vi "PEM SubVI.vi"(0 "VISA Refnum in":refnum<visa-resource-name>, 2 "Nuevo Retardo":dbl min=0.0 max=19999.900390625 step=0.10000000149011612 format="%.3f", 3 "Nueva Long. de Onda (nm)":dbl min=0.0 max=19999.9 step=0.1 format="%.1f", 5 "Cambiar Retardo PEM":bool, 7 "Cambiar L. Onda PEM":bool, 9 "Leer Frecuencia":bool, 11 "error in (no error)":errorcluster, 13 "Reiniciar Valores":bool, 14 "stop":bool) -> (4 "VISA Refnum out":refnum<visa-resource-name>, 6 "Longitud de onda (nm)":dbl format="%_5f", 8 "Retardo":dbl format="%_5f", 10 "Frecuencia":dbl format="%_5f", 15 "error out":errorcluster)   [LabVIEW 2016]
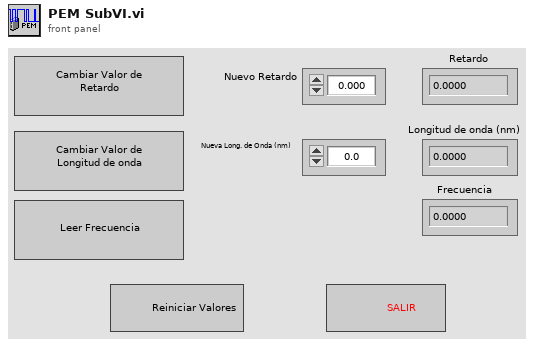
[diagram p1: front panel]
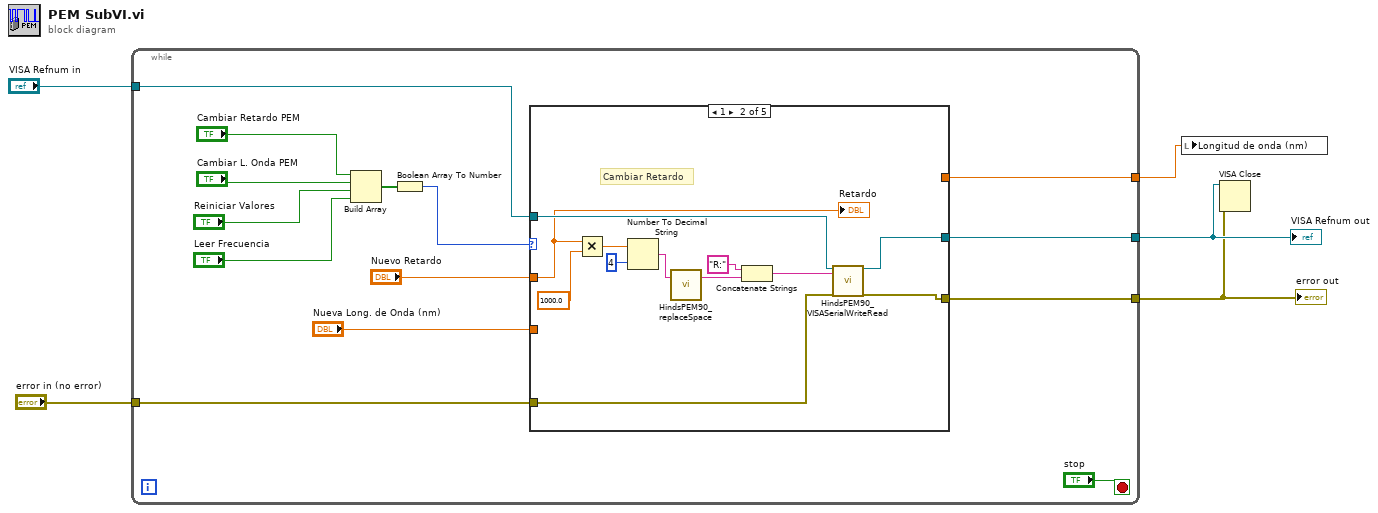
[diagram p0: block diagram]
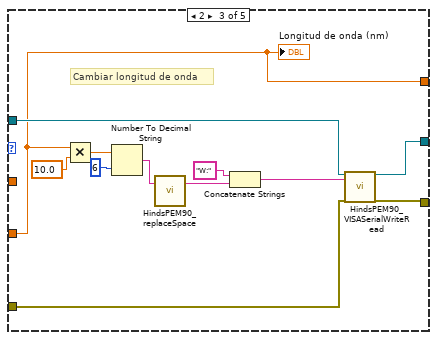
[diagram p3: hidden frame]
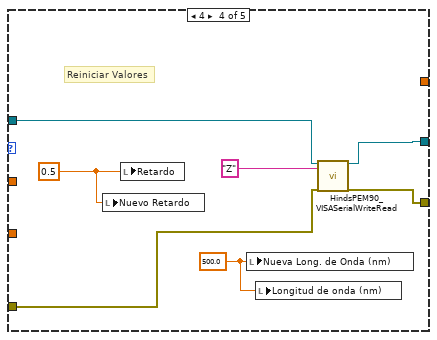
[diagram p4: hidden frame]
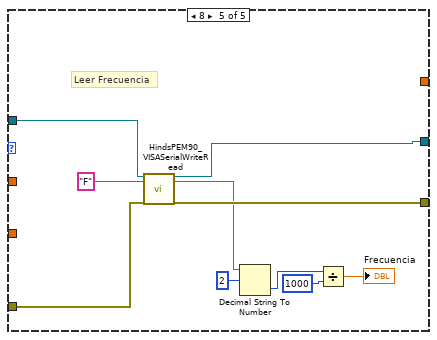
[diagram p5: hidden frame]
diagram:
  n1 = while {
    tunnel: "VISA Refnum in" -> [w10]
    tunnel: [w9] -> w3
    tunnel: [w8] -> w2
    tunnel: "error in (no error)" -> [w7]
    tunnel: [w6] -> w1
    stop <- "stop" stop-if-true
    n2 = Build Array("Cambiar Retardo PEM", "Cambiar L. Onda PEM", "Reiniciar Valores", "Leer Frecuencia") -> (w15:bool[])
    n3 = Boolean Array To Number(Boolean array=w15) -> (number=w16:u32)
    n4 = case shown="1" w16 {
      tunnel: "Nuevo Retardo" -> [_ w21 _ _ _]
      tunnel: "Nueva Long. de Onda (nm)" -> [_ _ w32 _ _]
      tunnel: [_ w23 w34 w47 w57] -> w8
      tunnel: w10 -> [_ w25 w37 w49 w59]
      tunnel: [_ w24 w36 w48 w58] -> w9
      tunnel: w7 -> [_ w20 w33 w44 w51]
      tunnel: [_ _ w32 _ _] -> w6
      frame 0, Default {
      }
      frame 1 {
        # "Cambiar Retardo"
        n5 = Multiply(x=w21, y=1000.0) -> (x*y=w28:dbl)
        n6 = Number To Decimal String(number=w28, width (-)=i16 4) -> (decimal integer string=w29:string)
        n7 = call "HindsPEM90_replaceSpace.vi"("Sting In"=w29) -> ("String Out"=w30:string)  [unwired: 17 in, 1 out]
        n8 = Concatenate Strings("R:" ("Substring"), w30) -> (w22:string)
        n9 = call "HindsPEM90_VISASerialWriteRead.vi"("VISA refnum in"=w25, "write"=w22, "error in (no error)"=w20) -> ("VISA refnum out"=w24:refnum<visa-resource-name>, "error out"=w23:errorcluster)  [unwired: 14 in, 1 out]
        "Retardo" <- w21
      }
      frame 2 {
        # "Cambiar longitud de onda"
        n10 = Multiply(x=w32, y=10.0) -> (x*y=w40:dbl)
        n11 = Number To Decimal String(number=w40, width (-)=i16 6) -> (decimal integer string=w43:string)
        n12 = call "HindsPEM90_replaceSpace.vi"("Sting In"=w43) -> ("String Out"=w42:string)  [unwired: 17 in, 1 out]
        n13 = Concatenate Strings("W:" ("Substring"), w42) -> (w35:string)
        n14 = call "HindsPEM90_VISASerialWriteRead.vi"("VISA refnum in"=w37, "write"=w35, "error in (no error)"=w33) -> ("VISA refnum out"=w36:refnum<visa-resource-name>, "error out"=w34:errorcluster)  [unwired: 14 in, 1 out]
        "Longitud de onda (nm)" <- w32
      }
      frame 4 {
        w45 = 500.0 ("Nueva Long. de Onda (nm)")
        w46 = 0.5 ("Retardo")
        # "Reiniciar Valores"
        n15 = local write "Nuevo Retardo"(w46) -> ()
        n16 = local write "Retardo"(w46) -> ()
        n17 = local write "Nueva Long. de Onda (nm)"(w45) -> ()
        n18 = local write "Longitud de onda (nm)"(w45) -> ()
        n19 = call "HindsPEM90_VISASerialWriteRead.vi"("VISA refnum in"=w49, "write"="Z", "error in (no error)"=w44) -> ("VISA refnum out"=w48:refnum<visa-resource-name>, "error out"=w47:errorcluster)  [unwired: 14 in, 1 out]
      }
      frame 8 {
        # "Leer Frecuencia"
        n20 = call "HindsPEM90_VISASerialWriteRead.vi"("VISA refnum in"=w59, "write"="F", "error in (no error)"=w51) -> ("VISA refnum out"=w58:refnum<visa-resource-name>, "read buffer"=w52:string, "error out"=w57:errorcluster)  [unwired: 14 in]
        n21 = Decimal String To Number(string=w52, offset=2) -> (number=w54:i32)  [unwired: 1 in, 1 out]
        n22 = Divide(x=w54, y=1000) -> (x/y=→"Frecuencia":dbl)
      }
    }
  }
  "error out" <- w2
  "VISA Refnum out" <- w3
  n23 = local write "Longitud de onda (nm)"(w1) -> ()
  n24 = VISA Close(VISA resource name=w3, error in (no error)=w2) -> ()  [unwired: 1 out]
